vi "Get IO Pin Counts.vi"(8 "error in (no error)":errorcluster, 9 "Device Number":string, 11 "VISA resource name":refnum<visa-resource-name>) -> (0 "error out":errorcluster, 1 "Digital Output Count":i32, 2 "Digital Input Count":i32, 3 "VISA resource name out":refnum<visa-resource-name>, 4 "Analog Output Count":i32, 5 "Analog Input Count":i32)   [LabVIEW 2018, in "Zaber A Series.lvlib"]
doc: "Detects the number of analog and digital input and output pins on a Zaber controller device.\n \nThis VI requires that the Initialize VI has been called with the same serial port."
uses:
  Zaber A Series.lvlib
  Private/All Commands.ctl
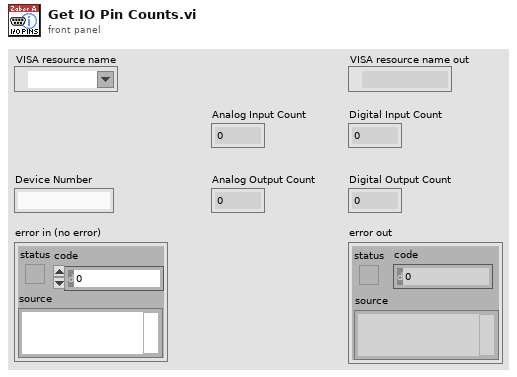
[diagram p1: front panel]
types:
  T1 = typedef "Zaber A Series.lvlib/All Commands.ctl" = string
  T2 = cluster{"Device":string, "Axis":string, "Reply Flag":string, "Status":string, "Warning Flags":string, "Data":string}
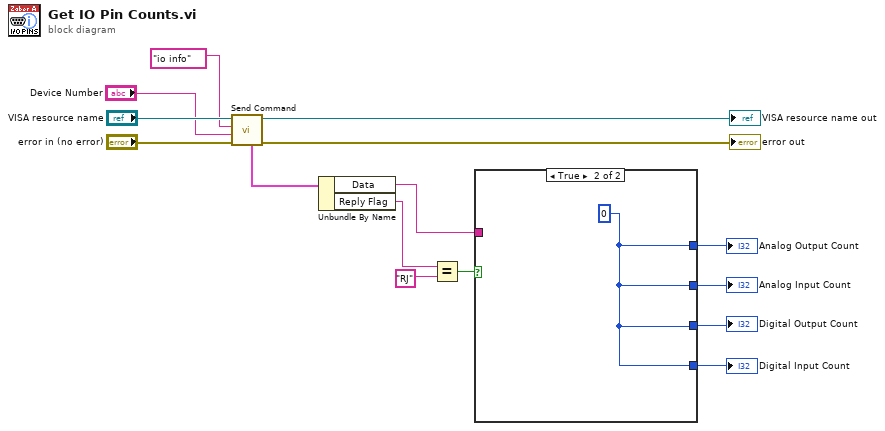
[diagram p0: block diagram]
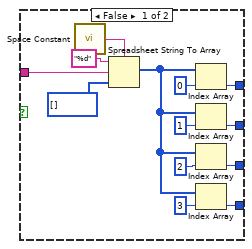
[diagram p2: hidden frame]
diagram:
  n1 = call "Send Command.vi"("error in (no error)"="error in (no error)", "Device and Axis"="Device Number", "Command"=T1 "io info" ("Complete Command List"), "VISA resource name"="VISA resource name") -> ("error out"=→"error out":errorcluster, "VISA resource name out"=→"VISA resource name out":refnum<visa-resource-name>, "First Response Bundle"=w1:T2)  [unwired: 2 in, 3 out]
  n2 = Unbundle By Name(w1) -> ("Data"=w3:string, "Reply Flag"=w2:string)
  n3 = Equal?(x=w2, y="RJ") -> (x = y?=w12:bool)
  n4 = case shown="True" w12 {
    tunnel: w3 -> [w20 _]
    tunnel: [w19 w29] -> w11
    tunnel: [w18 w29] -> w9
    tunnel: [w17 w29] -> w10
    tunnel: [w16 w29] -> w8
    frame False {
      n5 = call <vilib>:"Space Constant.vi"() -> ("String"=w28:string)
      n6 = Spreadsheet String To Array(delimiter (Tab)=w28, format string="%d", spreadsheet string=w20, array type (2D Dbl)=i32[] []) -> (array=w21:i32[])
      n7 = Index Array(array=w21, index=0) -> (element=w19:i32)
      n8 = Index Array(array=w21, index=1) -> (element=w17:i32)
      n9 = Index Array(array=w21, index=2) -> (element=w18:i32)
      n10 = Index Array(array=w21, index=3) -> (element=w16:i32)
    }
    frame True {
      w29 = 0
    }
  }
  "Analog Output Count" <- w11
  "Analog Input Count" <- w10
  "Digital Output Count" <- w9
  "Digital Input Count" <- w8
